vi "Accept.vi"(8 "error in (no error)":errorcluster, 10 "EquipmentVisitor":refnum<class "EquipmentVisitor.lvclass">, 11 "reference in":refnum<class "Rig.lvclass">) -> (0 "error out":errorcluster, 3 "reference in":refnum<class "Rig.lvclass">)   [LabVIEW 2020, in "Rig.lvclass"]
uses:
  Rig.lvclass
  EquipmentVisitor_class/EquipmentVisitor.lvclass
  Equipment_class/Equipment.lvclass
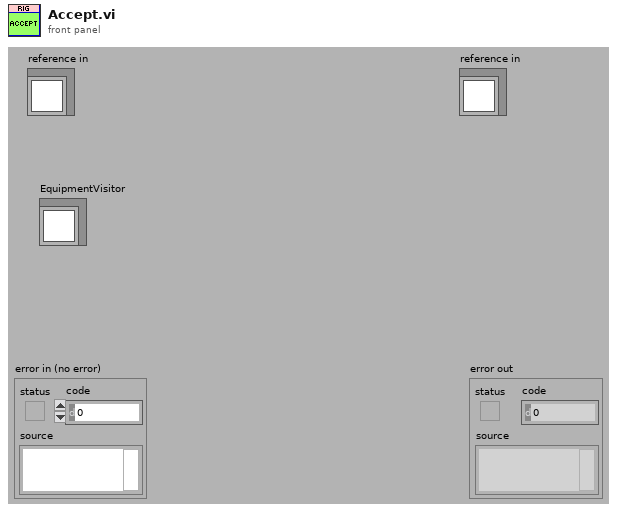
[diagram p1: front panel]
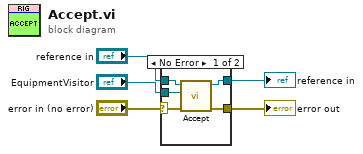
[diagram p0: block diagram]
diagram:
  n1 = case shown="No Error" "error in (no error)" {
    selector: "error in (no error)" -> [w8 w12]
    tunnel: [w7 w12] -> w4
    tunnel: [w6 w11] -> w2
    tunnel: "reference in" -> [w10 w11]
    tunnel: "EquipmentVisitor" -> [w9 _]
    frame No Error {
      n2 = call-parent "Accept.vi"("error in (no error)"=w8, "EquipmentVisitor"=w9, "reference in"=w10) -> ("error out"=w7:errorcluster, "reference out"=w6:refnum<class "Rig.lvclass">)  [unwired: 7 in]
    }
    frame Error {
    }
  }
  "error out" <- w4
  "reference in" <- w2
